vi "PIDControllers (SubVI).vi"(0 "HMI-10HIC200":dbl, 1 "HMI-10LIC200_MA":bool, 2 "BPCS-10LI200":dbl, 3 "HMI-10LIC200-SP":dbl, 5 "HMI-10LIC200-KPID":dbl[](array[numeric]), 7 "HMI-10TIC100-SP":dbl, 9 "BPCS-10TI100":dbl, 11 "HMI-10HIC300":dbl, 12 "HMI-10TIC100_MA":bool, 13 "HMI-10HIC100":dbl, 14 "HMI-10TIC100-KPID":dbl[](array[numeric]), 15 "BPCS-FJ":dbl) -> (4 "BPCS-10Y200":dbl format="%.2f", 6 "BPCS-SIM-TX-ARRAY":dbl[](array[numeric]), 8 "BPCS-10AY300":dbl, 10 "BPCS-10TY100":dbl format="%.2f")   [LabVIEW 2018]
uses:
  <vilib>/addons/control/pid/pid.llb/PID Advanced (DBL).vi
  <vilib>/addons/control/pid/NI_PID_pid.lvlib
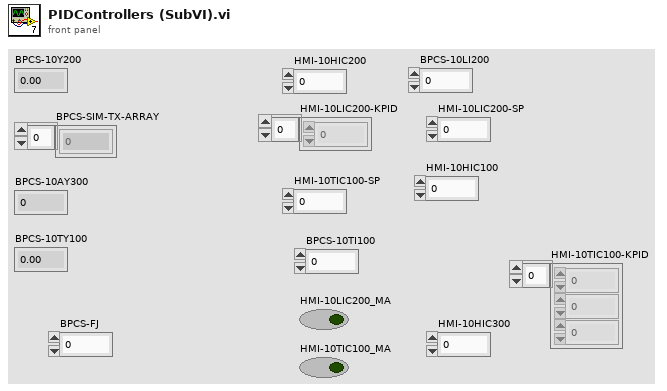
[diagram p1: front panel]
types:
  T1 = cluster{"proportional gain (Kc)":dbl, "integral time (Ti, min)":dbl, "derivative time (Td, min)":dbl}
  T2 = cluster{"HMI-10TIC100-KPID[0]":dbl, "HMI-10TIC100-KPID[1]":dbl, "HMI-10TIC100-KPID[2]":dbl}
  T3 = cluster{"HMI-10LIC200-KPID[0]":dbl, "HMI-10LIC200-KPID[1]":dbl, "HMI-10LIC200-KPID[2]":dbl}
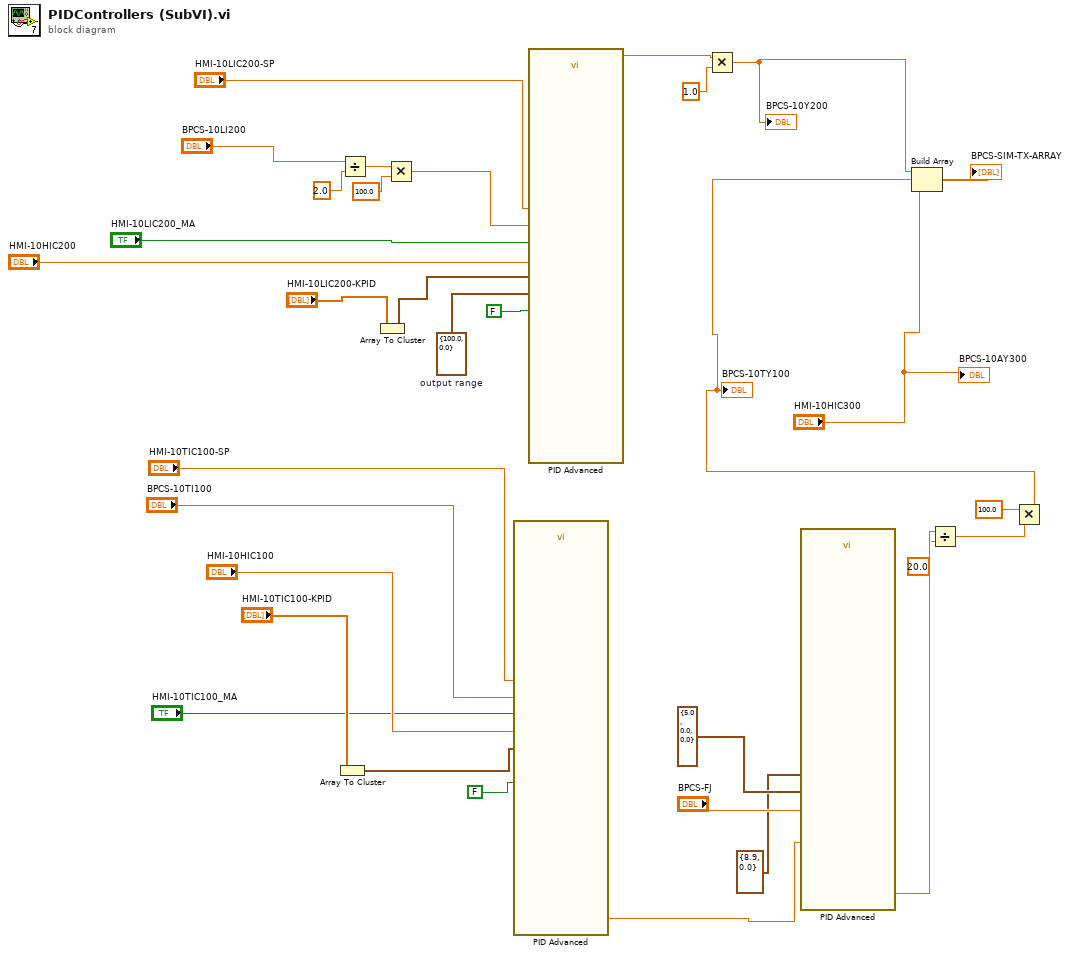
[diagram p0: block diagram]
diagram:
  w22 = cluster{"output high":dbl, "output low":dbl} {"output high"=100.0, "output low"=0.0}  # output range
  n1 = Array To Cluster(array="HMI-10TIC100-KPID") -> (cluster=w23:T2)
  n2 = Divide(x="BPCS-10LI200", y=2.0 ("x")) -> (x/y=w18:dbl)
  n3 = Array To Cluster(array="HMI-10LIC200-KPID") -> (cluster=w21:T3)
  n4 = Multiply(x=w18, y=100.0) -> (x*y=w20:dbl)
  n5 = call-poly <vilib>:"PID Advanced.vi"("setpoint"="HMI-10TIC100-SP", "auto? (T)"="HMI-10TIC100_MA", "manual control"="HMI-10HIC100", "process variable"="BPCS-10TI100", "PID gains"=w23, "reinitialize? (F)"=FALSE) -> ("output"=w4:dbl)  [unwired: 8 in, 1 out]
  n6 = call-poly <vilib>:"PID Advanced.vi"("setpoint"="HMI-10LIC200-SP", "output range"=w22, "auto? (T)"="HMI-10LIC200_MA", "manual control"="HMI-10HIC200", "process variable"=w20, "PID gains"=w21, "reinitialize? (F)"=FALSE) -> ("output"=w5:dbl)  [unwired: 7 in, 1 out]
  n7 = Multiply(x=w5, y=1.0 ("x")) -> (x*y=w6:dbl)
  "BPCS-10Y200" <- w6
  n8 = call-poly <vilib>:"PID Advanced.vi"("setpoint"=w4, "output range"=cluster{"setpoint high":dbl, "setpoint low":dbl} {"setpoint high"=8.9, "setpoint low"=0.0} ("setpoint range"), "process variable"="BPCS-FJ", "PID gains"=T1 {"proportional gain (Kc)"=5.0, "integral time (Ti, min)"=0.0, "derivative time (Td, min)"=0.0}) -> ("output"=w11:dbl)  [unwired: 10 in, 1 out]
  n9 = Divide(x=w11, y=20.0) -> (x/y=w12:dbl)
  n10 = Multiply(x=100.0, y=w12) -> (x*y=w9:dbl)
  "BPCS-10TY100" <- w9
  n11 = Build Array(w6, w9, "HMI-10HIC300") -> (→"BPCS-SIM-TX-ARRAY":dbl[])
  "BPCS-10AY300" <- "HMI-10HIC300"
